vi "UpdateCANData.vi"() -> ()   [LabVIEW 2011]
uses:
  _USB_CAN_T_R_Unit_.ctl
  <vilib>/Utility/miscctls.llb/LVRowAndColumnUnsignedTypeDef.ctl
  <vilib>/Utility/file.llb/Write To Spreadsheet File (string).vi
panel:
  in  "BuffLen":i32=200
  out "listcount":u32
  in  "open":bool
  in  "sPth_Sel":bool
  out "sv_pth":path
  in  "TSFormat":enum16{"原始值", "实际值"}(ring)
  in  "check2":bool
  in  "rate3":refnum<vi>
  in  "rate2":refnum<vi>
  in  "rate1":refnum<vi>
  in  "errcnt2":refnum<vi>
  in  "Trate2":bool
  in  "Trate1":bool
  in  "Rrate2":bool
  in  "Rrate1":bool
  in  "ForceUpt":bool
  in  "format":enum16{"hex", "dec", "oct", "bin"}(ring)
  in  "ID合并":bool
  in  "SaveCnt":refnum<vi>
  in  "path":refnum<vi>
  in  "rate0":refnum<vi>
  in  "vi ref":refnum<vi>
  in  "highspd":bool
  in  "cancelEvt":refnum<user-event>
  in  "check1":bool
  in  "errcnt1":refnum<vi>
  in  "save":bool
  in  "disp":bool=TRUE
  in  "stop":bool
  in  "savefile":bool
  in  "UseFilter":bool
  in  "Filter":u32[](array[numeric])
  in  "clear":bool
  in  "Enable":bool
  in  "list ref":refnum<vi>
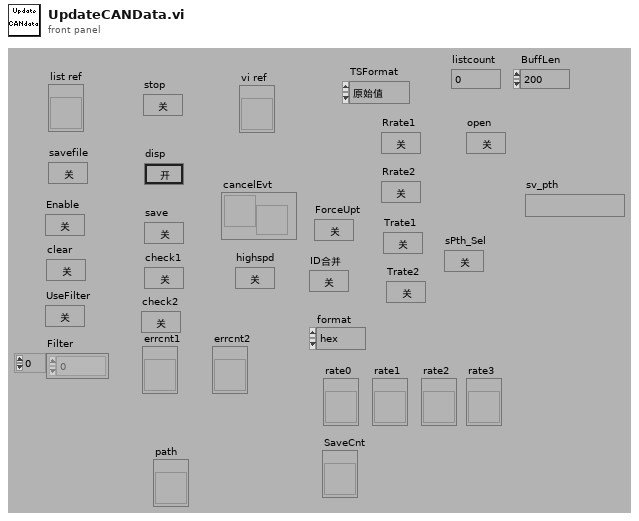
[diagram p1: front panel]
types:
  T1 = typedef "_USB_CAN_T_R_Unit_.ctl" = cluster{"time":timestamp, "channel":u16, "TimeStamp":u32, "tr":enum16{"接收", "发送"}, "id":u32, "Type":enum16{"数据帧", "远程帧"}, "Format":enum16{"标准帧", "扩展帧"}, "len":u8, "data":u8[], "sysTime":u32}
  T2 = typedef "LVRowAndColumnUnsignedTypeDef.ctl" = cluster{"Row":u32, "Column":u32}
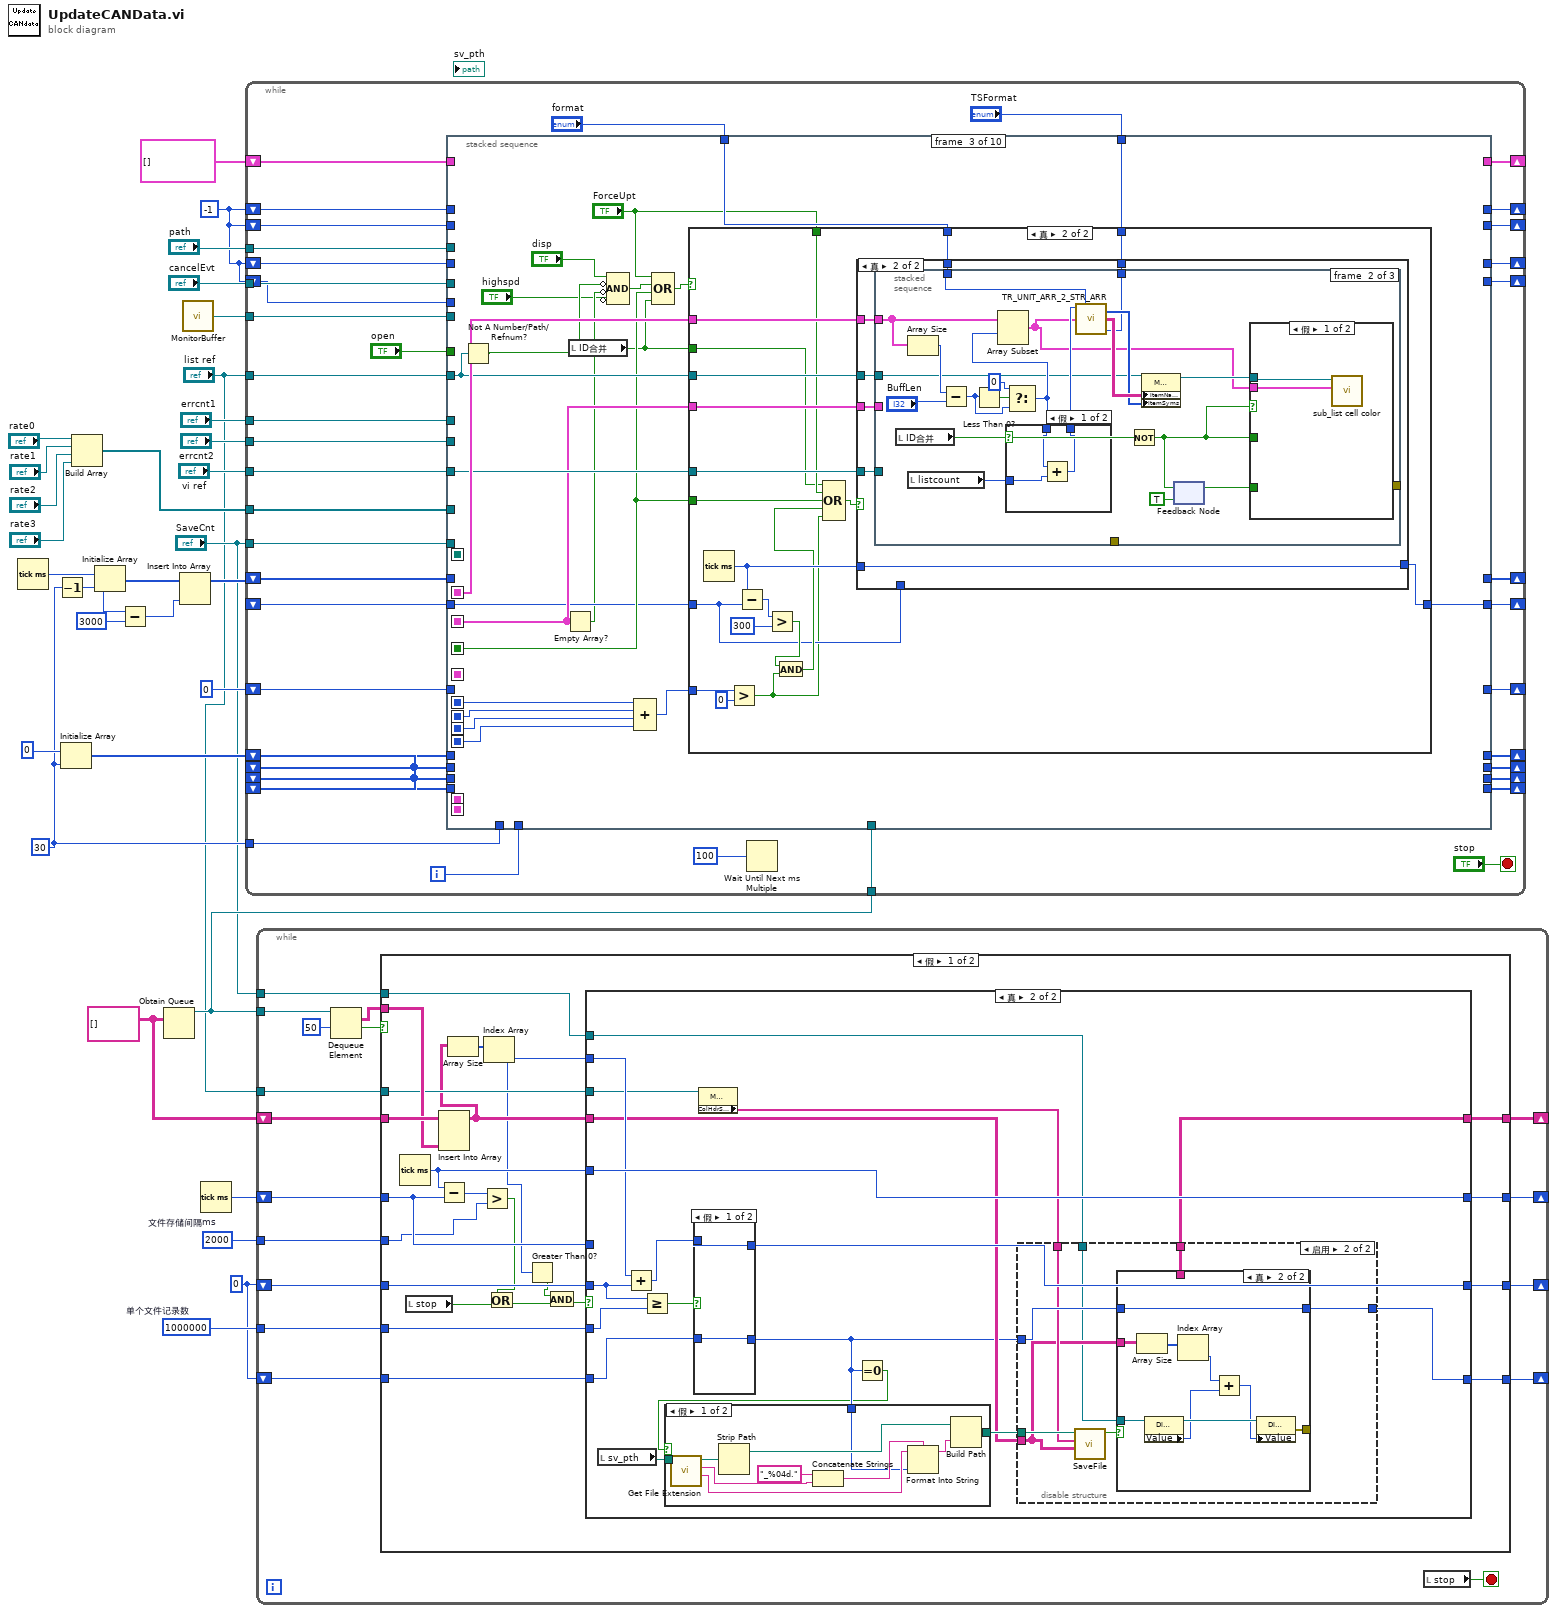
[diagram p0: block diagram]
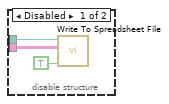
[diagram p4: hidden frame]
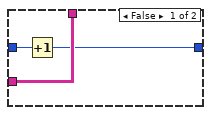
[diagram p5: hidden frame]
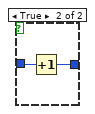
[diagram p6: hidden frame]
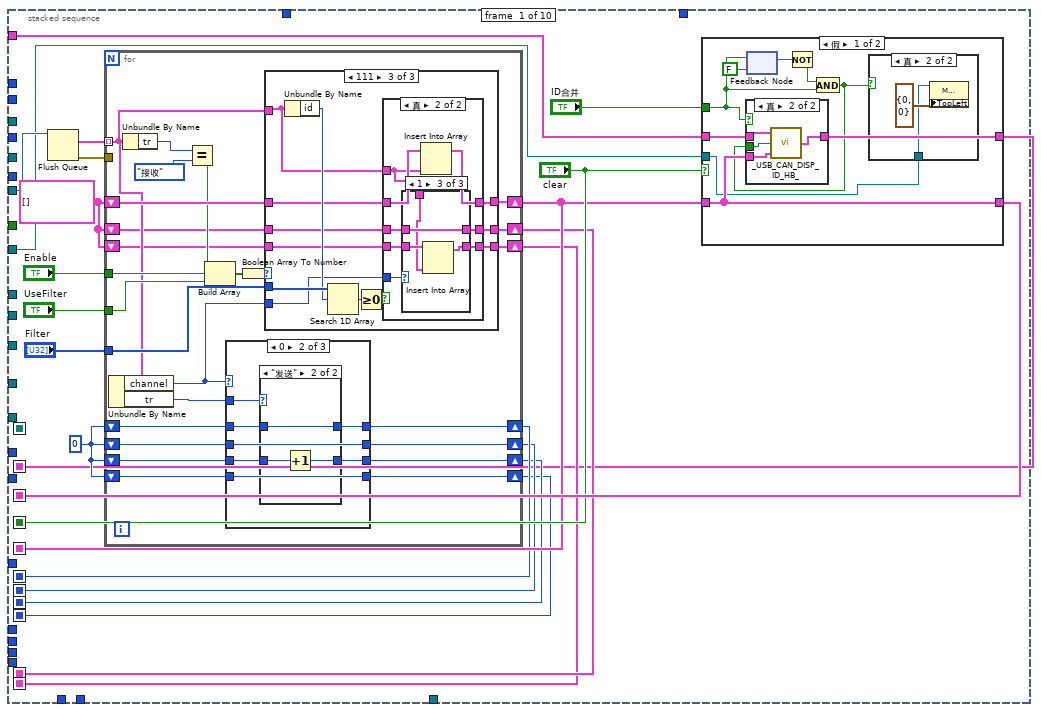
[diagram p8: hidden frame]
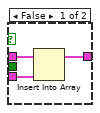
[diagram p9: hidden frame]
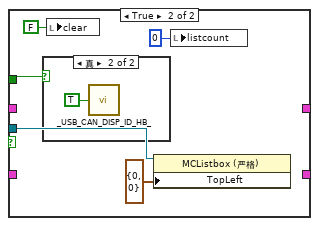
[diagram p11: hidden frame]
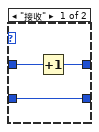
[diagram p14: hidden frame]
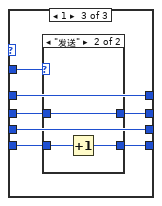
[diagram p15: hidden frame]
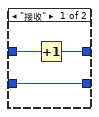
[diagram p16: hidden frame]
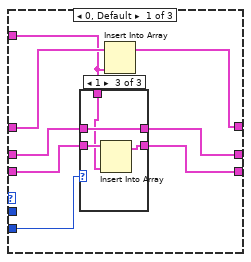
[diagram p17: hidden frame]
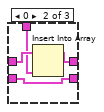
[diagram p19: hidden frame]
diagram:
  w5 = u32 2000  # 文件存储间隔ms
  w6 = 1000000  # 单个文件记录数
  w3 = 0
  w8 = string[][] [] ("strTable")
  w24 = 30 ("维数大小")
  w4 = i64 -1 ("U64")
  n1 = Tick Count (ms)() -> (millisecond timer value=w11:u32)
  n2 = Decrement(x=w24) -> (x-1=w23:i32)
  n3 = Initialize Array(0, w24) -> (w17:i32[])
  n4 = Build Array("rate0", "rate1", "rate2", "rate3") -> (w12:refnum<vi>[])
  n5 = Initialize Array(w11, w23) -> (w22:u32[])
  n6 = Subtract(x=w11, y=u32 3000) -> (x-y=w19:u32)
  n7 = Obtain Queue(element data type=w8) -> (queue out=w9:refnum<queue>)  [unwired: 4 in, 2 out]
  n8 = Insert Into Array(array=w22, new element=w19) -> (w21:u32[])  [unwired: 1 in]
  n9 = call "MonitorBuffer.vi"() -> ("USB_CAN_M_BUF"=w31:refnum<queue>)  [unwired: 1 in]
  n10 = Tick Count (ms)() -> (millisecond timer value=w7:u32)
  n11 = while {
    tunnel: w31 -> [w71]
    shift-right: [w69] -> _
    shift-left: T1[] [] -> [w70]
    tunnel: "list ref" -> [w68]
    shift-right: [w65] -> _
    shift-left: w4 -> [w67]
    tunnel: "errcnt1" -> [w66]
    tunnel: "cancelEvt" -> [w64]
    shift-right: [w62] -> _
    shift-left: 0 -> [w63]
    tunnel: "vi ref" -> [w61]
    shift-right: [w59] -> _
    shift-left: w17 -> [w60]
    tunnel: w24 -> [w57]
    tunnel: w12 -> [w56]
    shift-right: [w54] -> _
    shift-left: w21 -> [w55]
    tunnel: "SaveCnt" -> [w52]
    tunnel: "errcnt2" -> [w50]
    shift-right: [w46] -> _
    shift-left: w17 -> [w49]
    shift-right: [w45] -> _
    shift-left: w17 -> [w48]
    shift-right: [w44] -> _
    shift-left: w17 -> [w47]
    shift-right: [w42] -> _
    shift-left: w4 -> [w43]
    shift-right: [w40] -> _
    shift-left: _ -> [w41]
    tunnel: "path" -> [w38]
    tunnel: w9 -> [w37]
    shift-right: [w35] -> _
    shift-left: w4 -> [w36]
    shift-right: [w33] -> _
    shift-left: w4 -> [w34]
    i -> [w58]
    stop <- "stop" stop-if-true
    n12 = stacked-sequence {
      seq-local: [w73 _ _ _ _ _ _ _ _ _] -> [_ _ w319 _ _ w475 w510 _ _ _]
      seq-local: [w88 _ _ _ _ _ _ _ _ _] -> [_ _ w315 _ _ _ _ _ _ _]
      seq-local: [_ _ _ w394 _ _ _ _ _ _] -> [_ _ _ _ w450 _ _ _ _ _]
      seq-local: ["clear" _ _ _ _ _ _ _ _ _] -> [_ _ w312 _ _ _ _ _ _ _]
      seq-local: [w86 _ _ _ _ _ _ _ _ _] -> [_ _ _ _ w447 _ _ _ _ _]
      seq-local: [w82 _ _ _ _ _ _ _ _ _] -> [_ w249 w310 _ _ _ _ _ _ _]
      seq-local: [w81 _ _ _ _ _ _ _ _ _] -> [_ w237 w309 _ _ _ _ _ _ _]
      seq-local: [w80 _ _ _ _ _ _ _ _ _] -> [_ w236 w308 _ _ _ _ _ _ _]
      seq-local: [w79 _ _ _ _ _ _ _ _ _] -> [_ w235 w307 _ _ _ _ _ _ _]
      seq-local: [w77 _ _ _ _ _ _ _ _ _] -> [_ _ _ _ _ _ w519 w589 _ _]
      seq-local: [w76 _ _ _ _ _ _ _ _ _] -> [_ _ _ _ _ _ _ _ w632 w678]
      tunnel: w71 -> [w90 _ _ _ _ _ _ _ _ _]
      tunnel: w70 -> [w89 _ _ _ _ _ _ _ _ _]
      tunnel: [_ _ _ _ _ _ w512 _ _ _] -> w69
      tunnel: w68 -> [w74 _ w318 _ w449 w474 w511 _ _ _]
      tunnel: w67 -> [_ _ _ _ _ _ w520 _ _ _]
      tunnel: w66 -> [_ _ _ _ _ _ w517 _ _ _]
      tunnel: [_ _ _ _ _ _ w521 _ _ _] -> w65
      tunnel: w64 -> [_ _ _ _ w448 _ _ _ _ _]
      tunnel: w63 -> [_ _ _ _ w446 _ _ _ _ _]
      tunnel: [_ _ _ _ w445 _ _ _ _ _] -> w62
      tunnel: w61 -> [_ _ w316 w393 _ _ _ _ _ _]
      tunnel: w60 -> [_ w250 _ _ _ _ _ _ _ _]
      tunnel: [_ w248 _ _ _ _ _ _ _ _] -> w59
      tunnel: w58 -> [_ w244 _ _ _ _ _ _ _ _]
      tunnel: w57 -> [_ w251 _ _ _ _ _ _ _ _]
      tunnel: w56 -> [_ w231 _ _ _ _ _ _ _ _]
      tunnel: w55 -> [_ w247 _ _ _ _ _ _ _ _]
      tunnel: [_ w245 _ _ _ _ _ _ _ _] -> w54
      tunnel: w38 -> [_ _ _ w400 _ _ _ _ _ _]
      tunnel: w52 -> [_ _ _ w392 _ w473 _ _ _ _]
      tunnel: "format" -> [_ _ w314 _ w444 w472 _ _ _ _]
      tunnel: w50 -> [_ _ _ _ _ _ _ _ _ w677]
      tunnel: w49 -> [_ w241 _ _ _ _ _ _ _ _]
      tunnel: w48 -> [_ w240 _ _ _ _ _ _ _ _]
      tunnel: w47 -> [_ w239 _ _ _ _ _ _ _ _]
      tunnel: [_ w234 _ _ _ _ _ _ _ _] -> w46
      tunnel: [_ w233 _ _ _ _ _ _ _ _] -> w45
      tunnel: [_ w232 _ _ _ _ _ _ _ _] -> w44
      tunnel: w43 -> [_ _ _ _ _ _ _ _ _ w679]
      tunnel: [_ _ _ _ _ _ _ _ _ w680] -> w42
      tunnel: w41 -> [_ _ w311 _ _ _ _ _ _ _]
      tunnel: [_ _ w313 _ _ _ _ _ _ _] -> w40
      tunnel: "TSFormat" -> [_ _ w299 _ w441 _ _ _ _ _]
      tunnel: w37 -> [_ _ _ _ w440 _ _ _ _ _]
      tunnel: w36 -> [_ _ _ _ _ _ _ w588 _ _]
      tunnel: [_ _ _ _ _ _ _ w587 _ _] -> w35
      tunnel: w34 -> [_ _ _ _ _ _ _ _ w633 _]
      tunnel: [_ _ _ _ _ _ _ _ w631 _] -> w33
      tunnel: "open" -> [_ _ _ _ _ _ w516 w586 w630 w676]
      frame #0 {
        w83 = 0 ("和")
        w78 = T1[] []
        n13 = Flush Queue(queue=w90) -> (remaining elements=w85:T1[], error out=w75:errorcluster)  [unwired: 1 in, 1 out]
        n14 = for {
          tunnel: w85 -> [w132] mode=indexing
          shift-right: [w134] -> w86
          shift-left: w78 -> [w136]
          tunnel: "Enable" -> [w140]
          tunnel: "UseFilter" -> [w139]
          tunnel: "Filter" -> [w135]
          shift-right: [w126] -> w82
          shift-left: w83 -> [w130]
          shift-right: [w125] -> w81
          shift-left: w83 -> [w129]
          shift-right: [w124] -> w80
          shift-left: w83 -> [w128]
          shift-right: [w123] -> w79
          shift-left: w83 -> [w127]
          shift-right: [w120] -> w77
          shift-left: w78 -> [w122]
          shift-right: [w119] -> w76
          shift-left: w78 -> [w121]
          tunnel: w75 -> [_]
          n15 = Unbundle By Name(w132) -> ("channel"=w118:u16, "tr"=w131:enum16{"接收", "发送"})
          n16 = Unbundle By Name(w132) -> ("tr"=w142:enum16{"接收", "发送"})
          n17 = Equal?(x=w142, y=enum16{"接收", "发送"}."接收") -> (x = y?=w133:bool)
          n18 = Build Array(w133, w140, w139) -> (w138:bool[])
          n19 = case shown="0" w118 {
            tunnel: w131 -> [_ w153 w166]
            tunnel: w130 -> [w146 w151 w165]
            tunnel: w129 -> [w145 w148 w163]
            tunnel: w128 -> [w144 w149 w164]
            tunnel: w127 -> [w143 w152 w162]
            tunnel: [w146 w150 w165] -> w126
            tunnel: [w145 w148 w160] -> w125
            tunnel: [w144 w147 w164] -> w124
            tunnel: [w143 w152 w161] -> w123
            frame 255, Default {
            }
            frame 0 {
              n20 = case shown="\"发送\"" w153 {
                tunnel: w151 -> [w156 w159]
                tunnel: [w155 w159] -> w150
                tunnel: w149 -> [w154 w158]
                tunnel: [w154 w157] -> w147
                frame "接收" {
                  n21 = Increment(x=w156) -> (x+1=w155:i32)
                }
                frame "发送" {
                  n22 = Increment(x=w158) -> (x+1=w157:i32)
                }
              }
            }
            frame 1 {
              n23 = case shown="\"发送\"" w166 {
                tunnel: w163 -> [w169 w170]
                tunnel: w162 -> [w167 w172]
                tunnel: [w167 w171] -> w161
                tunnel: [w168 w170] -> w160
                frame "接收" {
                  n24 = Increment(x=w169) -> (x+1=w168:i32)
                }
                frame "发送" {
                  n25 = Increment(x=w172) -> (x+1=w171:i32)
                }
              }
            }
          }
          n26 = Boolean Array To Number(Boolean array=w138) -> (number=w137:u32)
          n27 = case shown="111" w137 {
            tunnel: w136 -> [w179 w193 w201]
            tunnel: w132 -> [w178 _ w200]
            tunnel: w135 -> [_ _ w205]
            tunnel: [w180 w193 w199] -> w134
            tunnel: w122 -> [w176 w192 w197]
            tunnel: w121 -> [w175 w191 w196]
            tunnel: [w174 w192 w195] -> w120
            tunnel: [w173 w191 w194] -> w119
            tunnel: w118 -> [w177 _ w198]
            frame 0, Default {
              n28 = case shown="1" w177 {
                tunnel: w176 -> [w182 w186 w190]
                tunnel: w175 -> [w181 w184 w188]
                tunnel: [w182 w185 w190] -> w174
                tunnel: [w181 w184 w189] -> w173
                tunnel: w178 -> [_ w183 w187]
                frame 255, Default {
                }
                frame 0 {
                  n29 = Insert Into Array(array=w186, new element=w183) -> (w185:T1[])  [unwired: 1 in]
                }
                frame 1 {
                  n30 = Insert Into Array(array=w188, new element=w187) -> (w189:T1[])  [unwired: 1 in]
                }
              }
              n31 = Insert Into Array(array=w179, new element=w178) -> (w180:T1[])  [unwired: 1 in]
            }
            frame 1, 5 {
            }
            frame 7 {
              n32 = Unbundle By Name(w200) -> ("id"=w204:u32)
              n33 = Search 1D Array(1D array=w205, element=w204) -> (index of element=w203:i32)  [unwired: 1 in]
              n34 = Greater Or Equal To 0?(x=w203) -> (x >= 0?=w202:bool)
              n35 = case shown="真" w202 {
                tunnel: w201 -> [w208 w216]
                tunnel: w200 -> [_ w209]
                tunnel: [w208 w215] -> w199
                tunnel: w198 -> [_ w214]
                tunnel: w197 -> [w207 w213]
                tunnel: w196 -> [w206 w212]
                tunnel: [w207 w211] -> w195
                tunnel: [w206 w210] -> w194
                frame False {
                }
                frame True {
                  n36 = case shown="1" w214 {
                    tunnel: w213 -> [w218 w222 w226]
                    tunnel: w212 -> [w217 w220 w224]
                    tunnel: [w218 w221 w226] -> w211
                    tunnel: [w217 w220 w225] -> w210
                    tunnel: w209 -> [_ w219 w223]
                    frame 255, Default {
                    }
                    frame 0 {
                      n37 = Insert Into Array(array=w222, new element=w219) -> (w221:T1[])  [unwired: 1 in]
                    }
                    frame 1 {
                      n38 = Insert Into Array(array=w224, new element=w223) -> (w225:T1[])  [unwired: 1 in]
                    }
                  }
                  n39 = Insert Into Array(array=w216, new element=w209) -> (w215:T1[])  [unwired: 1 in]
                }
              }
            }
          }
        }
        n40 = case shown="假" "clear" {
          tunnel: w86 -> [w102 _]
          tunnel: w89 -> [w101 _]
          tunnel: [w95 _] -> w73
          tunnel: [w102 _] -> w88
          tunnel: "ID合并" -> [w96 w112]
          tunnel: w74 -> [w97 w115]
          frame False {
            n41 = feedback-in #1(w96) -> ()
            n42 = feedback #1(FALSE ("ID合并")) -> (w99:bool)
            n43 = Not(x=w99) -> (.not. x?=w98:bool)
            n44 = And(x=w98, y=w96) -> (x .and. y?=w94:bool)
            n45 = case shown="真" w96 {
              tunnel: w102 -> [w105 w108]
              tunnel: w101 -> [w104 w109]
              tunnel: [w103 w107] -> w95
              tunnel: w94 -> [_ w106]
              frame False {
                n46 = Insert Into Array(array=w104, new element=w105) -> (w103:T1[])  [unwired: 1 in]
              }
              frame True {
                n47 = call "_USB_CAN_DISP_ID_HB_.vi"("arr new"=w108, "Reset buffer"=w106, "arr old"=w109) -> ("Arr Out"=w107:T1[])
              }
            }
            n48 = case shown="真" w94 {
              tunnel: w97 -> [_ w110]
              frame False {
              }
              frame True {
                n49 = property class="MCListbox (严格)"(reference=w110, "TopLeft"=T2 {"Row"=0, "Column"=0} ("左上可见单元格")) -> ()  [unwired: 1 in, 2 out]
              }
            }
          }
          frame True {
            n50 = case shown="真" w112 {
              frame False {
              }
              frame True {
                n51 = call "_USB_CAN_DISP_ID_HB_.vi"("Reset buffer"=TRUE) -> ()  [unwired: 2 in, 1 out]
              }
            }
            n52 = local write "clear"(FALSE ("clear")) -> ()
            n53 = property class="MCListbox (严格)"(reference=w115, "TopLeft"=T2 {"Row"=0, "Column"=0} ("左上可见单元格")) -> ()  [unwired: 1 in, 2 out]
            n54 = local write "listcount"(u32 0 ("listcount")) -> ()
          }
        }
      }
      frame #1 {
        n55 = Tick Count (ms)() -> (millisecond timer value=w246:u32)
        n56 = Quotient & Remainder(x=w244, y=w251) -> (x-y*floor(x/y)=w238:i32)  [unwired: 1 out]
        n57 = Replace Array Subset(array=w250, new element=w249, index=w238) -> (w248:i32[])
        n58 = Replace Array Subset(array=w241, new element=w237, index=w238) -> (w234:i32[])
        n59 = Replace Array Subset(array=w240, new element=w236, index=w238) -> (w233:i32[])
        n60 = Replace Array Subset(array=w239, new element=w235, index=w238) -> (w232:i32[])
        n61 = Replace Array Subset(array=w247, new element=w246, index=w238) -> (w245:u32[])
        n62 = Quotient & Remainder(x=w244, y=5) -> (x-y*floor(x/y)=w242:i32)  [unwired: 1 out]
        n63 = case shown="0" w242 {
          tunnel: w248 -> [_ w269]
          tunnel: w245 -> [_ w266]
          tunnel: w234 -> [_ w259]
          tunnel: w233 -> [_ w258]
          tunnel: w232 -> [_ w257]
          tunnel: w231 -> [_ w265]
          tunnel: "Rrate1" -> [_ w255]
          tunnel: "Rrate2" -> [_ w254]
          tunnel: "Trate1" -> [_ w253]
          tunnel: "Trate2" -> [_ w252]
          frame -1, Default {
          }
          frame 0 {
            w256 = 1000.0 ("y")
            n64 = Array Max & Min(array=w266) -> (max value=w268:u32, min value=w267:u32)  [unwired: 2 out]
            n65 = Subtract(x=w268, y=w267) -> (x-y=w260:u32)
            n66 = Index Array(array=w265) -> (element #1=w264:refnum<vi>, element #2=w263:refnum<vi>, element #3=w262:refnum<vi>, element #4=w261:refnum<vi>)  [unwired: 4 in]
            n67 = case shown="真" w255 {
              tunnel: w269 -> [_ w297]
              tunnel: w264 -> [_ w293]
              tunnel: w260 -> [_ w292]
              tunnel: w256 -> [_ w291]
              frame False {
              }
              frame True {
                n68 = Add Array Elements(numeric array=w297) -> (sum=w296:i32)
                n69 = Divide(x=w296, y=w292) -> (x/y=w295:dbl)
                n70 = Multiply(x=w295, y=w291) -> (x*y=w294:dbl)
                n71 = property class="DigNum (严格)"(reference=w293, "Value"=w294) -> ()  [unwired: 1 in, 2 out]
              }
            }
            n72 = case shown="真" w254 {
              tunnel: w263 -> [_ w287]
              tunnel: w260 -> [_ w286]
              tunnel: w259 -> [_ w285]
              tunnel: w256 -> [_ w284]
              frame False {
              }
              frame True {
                n73 = Add Array Elements(numeric array=w285) -> (sum=w288:i32)
                n74 = Divide(x=w288, y=w286) -> (x/y=w289:dbl)
                n75 = Multiply(x=w289, y=w284) -> (x*y=w290:dbl)
                n76 = property class="DigNum (严格)"(reference=w287, "Value"=w290) -> ()  [unwired: 1 in, 2 out]
              }
            }
            n77 = case shown="真" w253 {
              tunnel: w262 -> [_ w280]
              tunnel: w260 -> [_ w279]
              tunnel: w258 -> [_ w278]
              tunnel: w256 -> [_ w277]
              frame False {
              }
              frame True {
                n78 = Add Array Elements(numeric array=w278) -> (sum=w283:i32)
                n79 = Divide(x=w283, y=w279) -> (x/y=w282:dbl)
                n80 = Multiply(x=w282, y=w277) -> (x*y=w281:dbl)
                n81 = property class="DigNum (严格)"(reference=w280, "Value"=w281) -> ()  [unwired: 1 in, 2 out]
              }
            }
            n82 = case shown="真" w252 {
              tunnel: w261 -> [_ w273]
              tunnel: w260 -> [_ w272]
              tunnel: w257 -> [_ w271]
              tunnel: w256 -> [_ w270]
              frame False {
              }
              frame True {
                n83 = Add Array Elements(numeric array=w271) -> (sum=w274:i32)
                n84 = Divide(x=w274, y=w272) -> (x/y=w275:dbl)
                n85 = Multiply(x=w275, y=w270) -> (x*y=w276:dbl)
                n86 = property class="DigNum (严格)"(reference=w273, "Value"=w276) -> ()  [unwired: 1 in, 2 out]
              }
            }
          }
        }
      }
      frame #2 {
        n87 = Not A Number/Path/Refnum?(number/path/refnum=w318) -> (NaN/Path/Refnum?=w317:bool)
        n88 = Empty Array?(array=w315) -> (empty?=w305:bool)
        n89 = local read "ID合并"() -> (w298:bool)
        n90 = Compound Arithmetic op=AND("disp", invert w317, invert w305, invert "highspd") -> (w304:bool)
        n91 = Compound Arithmetic op=ADD(w310, w309, w308, w307) -> (w301:i32)
        n92 = Compound Arithmetic op=OR("ForceUpt", w304, w312, w298) -> (w303:bool)
        n93 = case shown="真" w303 {
          tunnel: w318 -> [_ w339]
          tunnel: w319 -> [_ w340]
          tunnel: w316 -> [_ w338]
          tunnel: w315 -> [_ w337]
          tunnel: w314 -> [_ w336]
          tunnel: w311 -> [w320 w324]
          tunnel: [w320 w335] -> w313
          tunnel: "ForceUpt" -> [_ w333]
          tunnel: w312 -> [_ w332]
          tunnel: w301 -> [_ w330]
          tunnel: w299 -> [_ w322]
          tunnel: w298 -> [_ w321]
          frame False {
          }
          frame True {
            n94 = Tick Count (ms)() -> (millisecond timer value=w331:u32)
            n95 = Greater?(x=w330, y=0) -> (0:w323:bool)
            n96 = Subtract(x=w331, y=w324) -> (x-y=w328:u32)
            n97 = Greater?(x=w328, y=u32 300) -> (0:w326:bool)
            n98 = And(x=w326, y=w323) -> (x .and. y?=w325:bool)
            n99 = Compound Arithmetic op=OR(w321, w333, w332, w325, w323) -> (w334:bool)
            n100 = case shown="真" w334 {
              tunnel: w340 -> [_ w348]
              tunnel: w339 -> [_ w347]
              tunnel: w338 -> [_ w346]
              tunnel: w337 -> [_ w345]
              tunnel: w336 -> [_ w344]
              tunnel: [w341 w343] -> w335
              tunnel: w331 -> [_ w343]
              tunnel: w324 -> [w341 _]
              tunnel: w322 -> [_ w342]
              frame False {
              }
              frame True {
                n101 = stacked-sequence {
                  tunnel: w348 -> [_ w355 _]
                  tunnel: w347 -> [_ w361 _]
                  tunnel: w346 -> [w353 _ w391]
                  tunnel: [w349 _ _] -> _
                  tunnel: [_ _ w387] -> _
                  tunnel: w345 -> [_ _ _]
                  tunnel: w344 -> [_ w371 _]
                  tunnel: w342 -> [_ w368 _]
                  frame #0 {
                    n102 = property class="VI"(reference=w353) -> (error out=w350:errorcluster, "Panel"=w352:refnum<vi>)  [unwired: 1 in, 1 out]
                    n103 = property class="Pnl"(reference=w352, error in=w350, "DeferPanUpdts"=TRUE ("延迟前面板更新")) -> (error out=w349:errorcluster)  [unwired: 1 out]
                  }
                  frame #1 {
                    n104 = local read "ID合并"() -> (w365:bool)
                    n105 = Array Size(array=w355) -> (size(s)=w370:i32)
                    n106 = local read "listcount"() -> (w362:u32)
                    n107 = Subtract(x=w370, y="BuffLen") -> (x-y=w369:i32)
                    n108 = Less Than 0?(x=w369) -> (x < 0?=w367:bool)
                    n109 = Select(t=0, s=w367, f=w369) -> (s? t:f=w364:i32)
                    n110 = Array Subset(array=w355, index=w364) -> (w359:T1[])  [unwired: 1 in]
                    n111 = case shown="假" w365 {
                      tunnel: w364 -> [w375 w377]
                      tunnel: [w374 w377] -> w363
                      tunnel: w362 -> [w376 _]
                      frame False {
                        n112 = Add(x=w375, y=w376) -> (x+y=w374:u32)
                      }
                      frame True {
                      }
                    }
                    n113 = call "TR_UNIT_ARR_2_STR_ARR.vi"("offset"=w363, "TR_Unit_Arr"=w359, "format"=w371, "TSFormat"=w368) -> ("smb"=w372:i32[], "strTable"=w373:string[][])  [unwired: 10 in]
                    n114 = Not(x=w365) -> (.not. x?=w358:bool)
                    n115 = property class="MCListbox (严格)"(reference=w361, "ItemNames"=w373, "ItemSyms"=w372) -> (reference out=w360:refnum<vi>)  [unwired: 1 in, 1 out]
                    n116 = feedback-in #2(w358) -> ()
                    n117 = feedback #2(TRUE) -> (w356:bool)
                    n118 = case shown="假" w358 {
                      tunnel: w360 -> [w379 w384]
                      tunnel: w358 -> [_ w383]
                      tunnel: w359 -> [w378 _]
                      tunnel: w356 -> [_ w382]
                      frame False {
                        n119 = call "sub_list cell color.vi"("TR_Unit_Arr"=w378, "list ref"=w379) -> ()  [unwired: 8 in, 2 out]
                      }
                      frame True {
                        n120 = Exclusive Or(1:w382, 2:w383) -> (0:w381:bool)
                        n121 = call "DispLastRow(MList).vi"("显示尾行"=w383, "MCListbox引用句柄"=w384) -> ("Ctl句柄输出"=w380:refnum<vi>)  [unwired: 8 in, 1 out]
                        n122 = case shown="真" w381 {
                          tunnel: w380 -> [_ w386]
                          frame False {
                          }
                          frame True {
                            n123 = call "sub_list cell color.vi"("Reset?(F)"=TRUE, "list ref"=w386) -> ()  [unwired: 8 in, 2 out]
                          }
                        }
                      }
                    }
                  }
                  frame #2 {
                    n124 = property class="VI"(reference=w391) -> (error out=w388:errorcluster, "Panel"=w390:refnum<vi>)  [unwired: 1 in, 1 out]
                    n125 = property class="Pnl"(reference=w390, error in=w388, "DeferPanUpdts"=FALSE ("延迟前面板更新")) -> (error out=w387:errorcluster)  [unwired: 1 out]
                  }
                }
              }
            }
          }
        }
      }
      frame #3 {
        n126 = local read "highspd"() -> (w399:bool)
        n127 = local read "sv_pth"() -> (w395:path)
        n128 = Not(x=w399) -> (.not. x?=w396:bool)
        n129 = And(x="save", y=w396) -> (x .and. y?=w397:bool)
        n130 = case shown="真" w397 {
          tunnel: w395 -> [w401 w408]
          tunnel: [w401 w411] -> w394
          tunnel: w400 -> [_ w410]
          tunnel: [_ w409] -> _
          tunnel: w393 -> [_ w403]
          tunnel: w392 -> [_ w402]
          frame False {
          }
          frame True {
            n131 = Not A Number/Path/Refnum?(number/path/refnum=w408) -> (NaN/Path/Refnum?=w407:bool)
            n132 = Empty String/Path?(string/path=w408) -> (empty?=w406:bool)
            n133 = Compound Arithmetic op=OR(w407, w406, "sPth_Sel") -> (w405:bool)
            n134 = case shown="真" w405 {
              tunnel: w408 -> [w412 _]
              tunnel: [w412 w422] -> w411
              tunnel: w403 -> [_ w418]
              tunnel: w402 -> [_ w415]
              frame False {
              }
              frame True {
                n135 = call "文件对话框"("prompt"="File Save As", "pattern (all files)"="*.csv", "pattern label"="Excel csv File") -> ("selected path"=w423:path, "exists"=w414:bool, "cancelled"=w424:bool, "error out"=w426:errorcluster)  [unwired: 9 in]
                n136 = Unbundle By Name(w426) -> ("status"=w425:bool)
                n137 = local write "sPth_Sel"(FALSE ("sPth_Sel")) -> ()
                n138 = case shown="真" w414 {
                  tunnel: [TRUE ("T button?") w437] -> w413
                  frame False {
                  }
                  frame True {
                    n139 = call "sub-Language-get str-const.vi"("sid"=u32 291) -> ("str"=w433:string)
                    n140 = call "sub-Language-get str-const.vi"("sid"=u32 268) -> ("str"=w431:string)
                    n141 = call "sub-Language-get str-const.vi"("sid"=u32 290) -> ("str"=w435:string)
                    n142 = Two Button Dialog(message=w435, 1:w431, 2:w433) -> (T button?=w437:bool)
                  }
                }
                n143 = Compound Arithmetic op=OR(invert w413, w424, w425) -> (w419:bool)
                n144 = Not(x=w419) -> (.not. x?=w416:bool)
                n145 = Select(t=path "", s=w419, f=w423) -> (s? t:f=w422:path)
                n146 = case shown="真" w416 {
                  tunnel: w415 -> [_ w439]
                  frame False {
                  }
                  frame True {
                    n147 = property class="DigNum (严格)"(reference=w439, "Value"=u32 0 ("值")) -> ()  [unwired: 1 in, 2 out]
                  }
                }
                n148 = invoke class="VI" method="Ctrl Val.Set"(reference=w418, "Control Name"="savefile" ("控件名"), "Value"=w416) -> ()  [unwired: 2 in, 5 out]
              }
            }
            n149 = property class="Path"(reference=w410, "Value"=w411) -> (error out=w409:errorcluster)  [unwired: 1 in, 1 out]
          }
        }
        n150 = local write "sv_pth"(w394) -> ()
      }
      frame #4 {
        n151 = local read "highspd"() -> (w443:bool)
        n152 = Not A Number/Path/Refnum?(number/path/refnum=w450) -> (NaN/Path/Refnum?=w454:bool)
        n153 = local read "save"() -> (w453:bool)
        n154 = Not(x=w454) -> (.not. x?=w452:bool)
        n155 = Not(x=w443) -> (.not. x?=w442:bool)
        n156 = Compound Arithmetic op=AND(w453, w452, w442) -> (w451:bool)
        n157 = case shown="真" w451 {
          tunnel: w447 -> [_ w470]
          tunnel: w450 -> [_ _]
          tunnel: w449 -> [_ _]
          tunnel: w448 -> [w457 _]
          tunnel: w446 -> [w455 w467]
          tunnel: [w455 w469] -> w445
          tunnel: w444 -> [_ w466]
          tunnel: w441 -> [_ w465]
          tunnel: w440 -> [_ w464]
          frame False {
            n158 = local read "save"() -> (w456:bool)
            n159 = case shown="真" w456 {
              tunnel: w457 -> [_ w460]
              frame False {
              }
              frame True {
                n160 = Generate User Event(user event=w460, event data cluster=FALSE ("事件数据")) -> (error out=w458:errorcluster)  [unwired: 1 in, 1 out]
                n161 = local write "save"(FALSE ("save")) -> ()
                n162 = call <vilib>:"Clear Errors.vi"("error in (no error)"=w458) -> ()  [unwired: 6 in, 1 out]
              }
            }
          }
          frame True {
            n163 = Array Size(array=w470) -> (size(s)=w468:i32)
            n164 = call "TR_UNIT_ARR_2_STR_ARR.vi"("offset"=w467, "TR_Unit_Arr"=w470, "format"=w466, "ForceString"=TRUE, "TSFormat"=w465) -> ("strTable"=w463:string[][])  [unwired: 9 in, 1 out]
            n165 = Add(x=w468, y=w467) -> (x+y=w469:i32)
            n166 = Enqueue Element(queue=w464, element=w463) -> ()  [unwired: 2 in, 3 out]
          }
        }
      }
      frame #5 {
        n167 = case shown="真" "savefile" {
          tunnel: w475 -> [_ w478]
          tunnel: w474 -> [_ w477]
          tunnel: w473 -> [_ _]
          tunnel: w472 -> [_ w476]
          frame False {
          }
          frame True {
            n168 = local write "savefile"(FALSE ("savefile")) -> ()
            n169 = call "文件对话框2"("prompt"="File Save As", "pattern (all files)"="*.csv", "pattern label"="Excel File") -> ("selected path"=w479:path, "exists"=w483:bool, "cancelled"=w484:bool, "error out"=w486:errorcluster)  [unwired: 9 in]
            n170 = Unbundle By Name(w486) -> ("status"=w485:bool)
            n171 = Not And(1:w485, 2:w484) -> (0:w481:bool)
            n172 = case shown="真" w483 {
              tunnel: [TRUE ("T button?") w508] -> w482
              frame False {
              }
              frame True {
                n173 = call "sub-Language-get str-const.vi"("sid"=u32 292) -> ("str"=w506:string)
                n174 = call "sub-Language-get str-const.vi"("sid"=u32 293) -> ("str"=w504:string)
                n175 = call "sub-Language-get str-const.vi"("sid"=u32 268) -> ("str"=w502:string)
                n176 = Two Button Dialog(message=w506, 1:w502, 2:w504) -> (T button?=w508:bool)
              }
            }
            n177 = And(x=w482, y=w481) -> (x .and. y?=w480:bool)
            n178 = case shown="真" w480 {
              tunnel: w479 -> [_ w498]
              tunnel: w478 -> [_ w493]
              tunnel: w477 -> [_ w499]
              tunnel: [_ w492] -> _
              tunnel: w476 -> [_ w491]
              frame False {
              }
              frame True {
                n179 = property class="MCListbox (严格)"(reference=w499) -> (error out=w500:errorcluster, "ColHdrString"=w496:string[])  [unwired: 1 in, 1 out]
                n180 = call "TR_UNIT_ARR_2_STR_ARR.vi"("TR_Unit_Arr"=w493, "format"=w491) -> ("strTable"=w494:string[][])  [unwired: 12 in, 1 out]
                n181 = call <vilib>:"Clear Errors.vi"("error in (no error)"=w500) -> ()  [unwired: 6 in, 1 out]
                n182 = Insert Into Array(array=w494, index (row)=0 ("索引 (行)"), new element=w496) -> (w495:string[][])  [unwired: 1 in]
                n183 = call-poly <vilib>:"Write To Spreadsheet File.vi"("2D data"=w495, "file path (dialog if empty)"=w498) -> ()  [unwired: 6 in, 1 out]
                n184 = Array Size(array=w493) -> (size(s)=w492:i32)
              }
            }
          }
        }
      }
      frame #6 {
        w509 = 99999 ("y")
        # "最大缓存10万条记录"
        n185 = And(x=w516, y="check1") -> (x .and. y?=w514:bool)
        n186 = Array Size(array=w510) -> (size(s)=w513:i32)
        n187 = case shown="真" w514 {
          tunnel: w519 -> [_ w542]
          tunnel: [i64 -1 ("U64") w535] -> w521
          tunnel: w520 -> [_ w540]
          tunnel: w517 -> [w534 w543]
          frame False {
            n188 = property class="DigNum (严格)"(reference=w534, "Value"=0 ("值")) -> (error out=w532:errorcluster)  [unwired: 1 in, 1 out]
            n189 = call <vilib>:"Clear Errors.vi"("error in (no error)"=w532) -> ()  [unwired: 6 in, 1 out]
          }
          frame True {
            n190 = for {
              tunnel: w542 -> [w564] mode=indexing
              shift-right: [w562] -> w535
              shift-left: w540 -> [w561]
              tunnel: [w560] -> w541
              tunnel: [w559] -> w539
              shift-right: [w556] -> w536
              shift-left: i64[] [] -> [w557]
              n191 = Unbundle By Name(w564) -> ("tr"=w558:enum16{"接收", "发送"}, "id"=w559:u32, "data"=w563:u8[], "time"=w560:timestamp)
              n192 = case shown="\"接收\", 默认" w558 {
                tunnel: w563 -> [w573 _]
                tunnel: [w574 w585] -> w562
                tunnel: w561 -> [w575 w585]
                tunnel: w557 -> [w577 w584]
                tunnel: [w576 w584] -> w556
                frame "接收", Default {
                  n193 = call "U8_Arr_To_I64.vi"("data"=w573) -> ("I64"=w574:i64)
                  n194 = Array Size(array=w573) -> (size(s)=w572:i32)
                  n195 = Subtract(x=w574, y=w575) -> (x-y=w569:i64)
                  n196 = Multiply(x=w572, y=-256) -> (x*y=w570:i32)
                  n197 = Equal?(x=i64 1, y=w569) -> (x = y?=w567:bool)
                  n198 = Increment(x=w570) -> (x+1=w568:i32)
                  n199 = Equal?(x=w569, y=w568) -> (x = y?=w566:bool)
                  n200 = Or(x=w567, y=w566) -> (x .or. y?=w565:bool)
                  n201 = case shown="假" w565 {
                    tunnel: w577 -> [w582 w583]
                    tunnel: [w581 w583] -> w576
                    tunnel: w575 -> [w580 _]
                    tunnel: w574 -> [w579 _]
                    frame False {
                      n202 = Insert Into Array(array=w582, new element #1=w580, new element #2=w579) -> (w581:i64[])  [unwired: 1 in]
                    }
                    frame True {
                    }
                  }
                }
                frame "发送" {
                }
              }
            }
            n203 = Empty Array?(array=w536) -> (empty?=w537:bool)
            n204 = case shown="假" w537 {
              tunnel: w543 -> [w555 _]
              tunnel: w541 -> [w551 _]
              tunnel: w539 -> [w550 _]
              tunnel: w536 -> [w547 _]
              frame False {
                n205 = property class="DigNum (严格)"(reference=w555) -> (reference out=w554:refnum<vi>, error out=w553:errorcluster, "Value"=w549:i32)  [unwired: 1 in]
                n206 = Array Size(array=w547) -> (size(s)=w546:i32)
                n207 = Divide(x=w546, y=2) -> (x/y=w544:dbl)
                n208 = Add(x=w549, y=w544) -> (x+y=w548:dbl)
                n209 = call "_USB_CAN_DEBUG_LOG_OUT_.vi"("id"=w550, "Edata"=w547, "TIME"=w551) -> ()  [unwired: 9 in]
                n210 = property class="DigNum (严格)"(reference=w554, error in=w553, "Value"=w548) -> (error out=w552:errorcluster)  [unwired: 1 out]
                n211 = call <vilib>:"Clear Errors.vi"("error in (no error)"=w552) -> ()  [unwired: 6 in, 1 out]
              }
              frame True {
              }
            }
          }
        }
        n212 = Greater?(x=w513, y=w509) -> (0:w518:bool)
        n213 = case shown="真" w518 {
          tunnel: w513 -> [_ w528]
          tunnel: w510 -> [w522 w526]
          tunnel: [w522 w524] -> w512
          tunnel: w511 -> [_ _]
          tunnel: w509 -> [_ w527]
          frame False {
          }
          frame True {
            n214 = Subtract(x=w528, y=w527) -> (x-y=w523:i32)
            n215 = local read "listcount"() -> (w530:u32)
            n216 = Delete From Array(array=w526, length=w523, index=0 ("索引")) -> (array with subset deleted=w524:T1[])  [unwired: 1 out]
            n217 = Compound Arithmetic op=ADD(w530, w523) -> (→"listcount":u32)
          }
        }
      }
      frame #7 {
        n218 = case shown="真" w586 {
          tunnel: w589 -> [_ w598]
          tunnel: w588 -> [w590 w592]
          tunnel: [w590 w591] -> w587
          frame False {
          }
          frame True {
            n219 = for {
              tunnel: w598 -> [w617] mode=indexing
              shift-right: [w615] -> w591
              shift-left: w592 -> [w614]
              tunnel: [w613] -> w597
              tunnel: [w609] -> w596
              shift-right: [w610] -> w593
              shift-left: i64[] [] -> [w611]
              n220 = Unbundle By Name(w617) -> ("tr"=w612:enum16{"接收", "发送"}, "id"=w609:u32, "TimeStamp"=w616:u32, "time"=w613:timestamp)
              n221 = case shown="\"接收\", 默认" w612 {
                tunnel: w616 -> [w619 _]
                tunnel: [w619 w629] -> w615
                tunnel: w614 -> [w620 w629]
                tunnel: w611 -> [w622 w628]
                tunnel: [w621 w628] -> w610
                tunnel: w609 -> [_ _]
                frame "接收", Default {
                  n222 = Greater?(x=w620, y=w619) -> (0:w618:bool)
                  n223 = case shown="真" w618 {
                    tunnel: w622 -> [w623 w627]
                    tunnel: [w623 w626] -> w621
                    tunnel: w620 -> [_ w625]
                    tunnel: w619 -> [_ w624]
                    frame False {
                    }
                    frame True {
                      n224 = Insert Into Array(array=w627, new element #1=w625, new element #2=w624) -> (w626:i64[])  [unwired: 1 in]
                    }
                  }
                }
                frame "发送" {
                }
              }
            }
            n225 = Empty Array?(array=w593) -> (empty?=w594:bool)
            n226 = case shown="假" w594 {
              tunnel: w597 -> [w608 _]
              tunnel: w596 -> [w607 _]
              tunnel: w593 -> [w606 _]
              frame False {
                n227 = call "sub-Language-get str-const.vi"("sid"=u32 294) -> ("str"=w604:string)
                n228 = call "sub-Language-get str-const.vi"("sid"=u32 295) -> ("str"=w601:string)
                n229 = Concatenate Strings(w604, ",ch1," ("字符串"), w601, ":" ("字符串")) -> (w599:string)
                n230 = call "_USB_CAN_DEBUG_LOG_OUT_.vi"("id"=w607, "Info"=w599, "Edata"=w606, "TIME"=w608) -> ()  [unwired: 8 in]
              }
              frame True {
              }
            }
          }
        }
      }
      frame #8 {
        n231 = case shown="真" w630 {
          tunnel: w633 -> [w634 w637]
          tunnel: w632 -> [_ w636]
          tunnel: [w634 w635] -> w631
          frame False {
          }
          frame True {
            n232 = for {
              tunnel: w636 -> [w661] mode=indexing
              shift-right: [w659] -> w635
              shift-left: w637 -> [w658]
              tunnel: [w657] -> w642
              tunnel: [w653] -> w641
              shift-right: [w654] -> w638
              shift-left: i64[] [] -> [w655]
              n233 = Unbundle By Name(w661) -> ("tr"=w656:enum16{"接收", "发送"}, "id"=w653:u32, "TimeStamp"=w660:u32, "time"=w657:timestamp)
              n234 = case shown="\"接收\", 默认" w656 {
                tunnel: w660 -> [w663 _]
                tunnel: [w663 w673] -> w659
                tunnel: w658 -> [w664 w673]
                tunnel: w655 -> [w666 w672]
                tunnel: [w665 w672] -> w654
                tunnel: w653 -> [_ _]
                frame "接收", Default {
                  n235 = Greater?(x=w664, y=w663) -> (0:w662:bool)
                  n236 = case shown="真" w662 {
                    tunnel: w666 -> [w667 w671]
                    tunnel: [w667 w670] -> w665
                    tunnel: w664 -> [_ w669]
                    tunnel: w663 -> [_ w668]
                    frame False {
                    }
                    frame True {
                      n237 = Insert Into Array(array=w671, new element #1=w669, new element #2=w668) -> (w670:i64[])  [unwired: 1 in]
                    }
                  }
                }
                frame "发送" {
                }
              }
            }
            n238 = Empty Array?(array=w638) -> (empty?=w639:bool)
            n239 = case shown="假" w639 {
              tunnel: w642 -> [w652 _]
              tunnel: w641 -> [w651 _]
              tunnel: w638 -> [w650 _]
              frame False {
                n240 = call "sub-Language-get str-const.vi"("sid"=u32 294) -> ("str"=w648:string)
                n241 = call "sub-Language-get str-const.vi"("sid"=u32 295) -> ("str"=w645:string)
                n242 = Concatenate Strings(w648, ",ch2," ("字符串"), w645, ":" ("字符串")) -> (w643:string)
                n243 = call "_USB_CAN_DEBUG_LOG_OUT_.vi"("id"=w651, "Info"=w643, "Edata"=w650, "TIME"=w652) -> ()  [unwired: 8 in]
              }
              frame True {
              }
            }
          }
        }
      }
      frame #9 {
        n244 = And(x=w676, y="check2") -> (x .and. y?=w674:bool)
        n245 = case shown="真" w674 {
          tunnel: w678 -> [_ w692]
          tunnel: [i64 -1 ("U64") w685] -> w680
          tunnel: w679 -> [_ w690]
          tunnel: w677 -> [w684 w693]
          frame False {
            n246 = property class="DigNum (严格)"(reference=w684, "Value"=0 ("值")) -> (error out=w682:errorcluster)  [unwired: 1 in, 1 out]
            n247 = call <vilib>:"Clear Errors.vi"("error in (no error)"=w682) -> ()  [unwired: 6 in, 1 out]
          }
          frame True {
            n248 = for {
              tunnel: w692 -> [w714] mode=indexing
              shift-right: [w712] -> w685
              shift-left: w690 -> [w711]
              tunnel: [w710] -> w691
              tunnel: [w709] -> w689
              shift-right: [w706] -> w686
              shift-left: i64[] [] -> [w707]
              n249 = Unbundle By Name(w714) -> ("tr"=w708:enum16{"接收", "发送"}, "id"=w709:u32, "data"=w713:u8[], "time"=w710:timestamp)
              n250 = case shown="\"接收\", 默认" w708 {
                tunnel: w713 -> [w723 _]
                tunnel: [w724 w735] -> w712
                tunnel: w711 -> [w725 w735]
                tunnel: w707 -> [w727 w734]
                tunnel: [w726 w734] -> w706
                frame "接收", Default {
                  n251 = call "U8_Arr_To_I64.vi"("data"=w723) -> ("I64"=w724:i64)
                  n252 = Array Size(array=w723) -> (size(s)=w722:i32)
                  n253 = Subtract(x=w724, y=w725) -> (x-y=w719:i64)
                  n254 = Multiply(x=w722, y=-256) -> (x*y=w720:i32)
                  n255 = Increment(x=w720) -> (x+1=w718:i32)
                  n256 = Equal?(x=w719, y=w718) -> (x = y?=w716:bool)
                  n257 = Equal?(x=i64 1, y=w719) -> (x = y?=w717:bool)
                  n258 = Or(x=w717, y=w716) -> (x .or. y?=w715:bool)
                  n259 = case shown="假" w715 {
                    tunnel: w727 -> [w732 w733]
                    tunnel: [w731 w733] -> w726
                    tunnel: w725 -> [w730 _]
                    tunnel: w724 -> [w729 _]
                    frame False {
                      n260 = Insert Into Array(array=w732, new element #1=w730, new element #2=w729) -> (w731:i64[])  [unwired: 1 in]
                    }
                    frame True {
                    }
                  }
                }
                frame "发送" {
                }
              }
            }
            n261 = Empty Array?(array=w686) -> (empty?=w687:bool)
            n262 = case shown="假" w687 {
              tunnel: w693 -> [w705 _]
              tunnel: w691 -> [w701 _]
              tunnel: w689 -> [w700 _]
              tunnel: w686 -> [w697 _]
              frame False {
                n263 = property class="DigNum (严格)"(reference=w705) -> (reference out=w704:refnum<vi>, error out=w703:errorcluster, "Value"=w699:i32)  [unwired: 1 in]
                n264 = Array Size(array=w697) -> (size(s)=w696:i32)
                n265 = Divide(x=w696, y=2) -> (x/y=w694:dbl)
                n266 = Add(x=w699, y=w694) -> (x+y=w698:dbl)
                n267 = call "_USB_CAN_DEBUG_LOG_OUT_.vi"("id"=w700, "Edata"=w697, "TIME"=w701) -> ()  [unwired: 9 in]
                n268 = property class="DigNum (严格)"(reference=w704, error in=w703, "Value"=w698) -> (error out=w702:errorcluster)  [unwired: 1 out]
                n269 = call <vilib>:"Clear Errors.vi"("error in (no error)"=w702) -> ()  [unwired: 6 in, 1 out]
              }
              frame True {
              }
            }
          }
        }
      }
    }
    n270 = Wait Until Next ms Multiple(millisecond multiple=u32 100 ("毫秒倍数")) -> ()  [unwired: 1 out]
  }
  n271 = while {
    tunnel: w9 -> [w751]
    shift-right: [w746] -> _
    shift-left: w8 -> [w747]
    tunnel: "list ref" -> [w745]
    shift-right: [w743] -> _
    shift-left: w7 -> [w744]
    shift-right: [w741] -> _
    shift-left: w3 -> [w742]
    tunnel: w6 -> [w740]
    tunnel: w5 -> [w739]
    shift-right: [w737] -> _
    shift-left: w3 -> [w738]
    tunnel: "SaveCnt" -> [w736]
    stop <- w752 stop-if-true
    n272 = Dequeue Element(queue=w751, timeout in ms (-1)=50 ("超时毫秒(-1)")) -> (element=w748:string[][], timed out?=w749:bool)  [unwired: 1 in, 2 out]
    n273 = case shown="假" w749 {
      tunnel: w748 -> [w774 _]
      tunnel: w747 -> [w775 w839]
      tunnel: [w766 w839] -> w746
      tunnel: w745 -> [w769 _]
      tunnel: w744 -> [w771 w838]
      tunnel: [w770 w838] -> w743
      tunnel: w742 -> [w768 w837]
      tunnel: [w767 w837] -> w741
      tunnel: w740 -> [w763 _]
      tunnel: w739 -> [w762 _]
      tunnel: w738 -> [w755 w836]
      tunnel: [w754 w836] -> w737
      tunnel: w736 -> [w753 _]
      frame False {
        n274 = Tick Count (ms)() -> (millisecond timer value=w772:u32)
        n275 = local read "stop"() -> (w764:bool)
        n276 = Insert Into Array(array=w775, new element=w774) -> (w760:string[][])  [unwired: 2 in]
        n277 = Subtract(x=w772, y=w771) -> (x-y=w773:u32)
        n278 = Array Size(array=w760) -> (size(s)=w761:i32[])
        n279 = Greater?(x=w773, y=w762) -> (0:w765:bool)
        n280 = Index Array(array=w761) -> (element=w756:i32)  [unwired: 1 in]
        n281 = Or(x=w765, y=w764) -> (x .or. y?=w759:bool)
        n282 = Greater Than 0?(x=w756) -> (x > 0?=w757:bool)
        n283 = And(x=w757, y=w759) -> (x .and. y?=w758:bool)
        n284 = case shown="真" w758 {
          tunnel: w772 -> [_ w797]
          tunnel: w771 -> [w779 _]
          tunnel: [w779 w797] -> w770
          tunnel: w769 -> [_ w781]
          tunnel: w768 -> [w778 w792]
          tunnel: [w778 w790] -> w767
          tunnel: w760 -> [w777 w785]
          tunnel: [w777 w788] -> w766
          tunnel: w763 -> [_ w794]
          tunnel: w756 -> [_ w795]
          tunnel: w755 -> [w776 w786]
          tunnel: [w776 w787] -> w754
          tunnel: w753 -> [_ w782]
          frame False {
          }
          frame True {
            n285 = local read "sv_pth"() -> (w796:path)
            n286 = Add(x=w795, y=w792) -> (x+y=w791:i32)
            n287 = Greater Or Equal?(x=w792, y=w794) -> (x >= y?=w789:bool)
            n288 = case shown="假" w789 {
              tunnel: w786 -> [w832 w835]
              tunnel: [w832 w834] -> w784
              tunnel: w791 -> [w833 _]
              tunnel: [w833 _] -> w790
              frame False {
              }
              frame True {
                n289 = Increment(x=w835) -> (x+1=w834:i32)
              }
            }
            n290 = property class="MCListbox (严格)"(reference=w781) -> ("ColHdrString"=w780:string[])  [unwired: 1 in, 2 out]
            n291 = Equal To 0?(x=w784) -> (x = 0?=w783:bool)
            n292 = case shown="假" w783 {
              tunnel: w796 -> [w804 w808]
              tunnel: [w799 w808] -> w793
              tunnel: w784 -> [w798 _]
              frame False {
                n293 = call <vilib>:"Get File Extension.vi"("file"=w804) -> ("filename without extension"=w803:string, "lowercase file extension"=w806:string, "dup file"=w805:path)  [unwired: 7 in, 1 out]
                n294 = Strip Path(path=w805) -> (stripped path=w801:path)  [unwired: 1 out]
                n295 = Concatenate Strings("_%04d." ("字符串"), w806) -> (w802:string)
                n296 = Format Into String(format string=w802, initial string=w803, w798) -> (resulting string=w800:string)  [unwired: 1 in, 1 out]
                n297 = Build Path(base path=w801, name or relative path=w800) -> (appended path=w799:path)
              }
              frame True {
              }
            }
            n298 = disable-structure shown="启用" {
              disable-tunnel: w785 -> [w811 w814]
              disable-tunnel: w793 -> [w809 w816]
              disable-tunnel: [_ w819] -> w788
              disable-tunnel: w784 -> [_ w818]
              disable-tunnel: [_ w817] -> w787
              disable-tunnel: w780 -> [_ w815]
              disable-tunnel: w782 -> [_ w812]
              frame Disabled {
                n299 = call-poly <vilib>:"Write To Spreadsheet File.vi"("append to file? (new file:F)"=TRUE, "2D data"=w811, "file path (dialog if empty)"=w809) -> ()  [unwired: 5 in, 1 out]
              }
              frame Enabled {
                n300 = call "SaveFile.vi"("数据"=w814, "文件头"=w815, "文件路径"=w816) -> ("Success"=w813:bool)  [unwired: 8 in]
                n301 = case shown="真" w813 {
                  tunnel: w814 -> [w822 w828]
                  tunnel: [w822 _] -> w819
                  tunnel: w818 -> [w821 w831]
                  tunnel: [w820 w831] -> w817
                  tunnel: w812 -> [_ w830]
                  tunnel: [_ w823] -> _
                  frame False {
                    n302 = Increment(x=w821) -> (x+1=w820:i32)
                  }
                  frame True {
                    n303 = Array Size(array=w828) -> (size(s)=w827:i32[])
                    n304 = property class="DigNum (严格)"(reference=w830) -> (reference out=w829:refnum<vi>, "Value"=w825:u32)  [unwired: 1 in, 1 out]
                    n305 = Index Array(array=w827) -> (element=w826:i32)  [unwired: 1 in]
                    n306 = Add(x=w826, y=w825) -> (x+y=w824:u32)
                    n307 = property class="DigNum (严格)"(reference=w829, "Value"=w824) -> (error out=w823:errorcluster)  [unwired: 1 in, 1 out]
                  }
                }
              }
            }
          }
        }
      }
      frame True {
      }
    }
    n308 = local read "stop"() -> (w752:bool)
  }
